vi "ExecuteState.vi"(0 "JSONRPC Server in":refnum<class "JSONRPC Server.lvclass">, 1 "IFw session":refnum<class "niInstr FIFO Register Bus v1 Host.lvclass">, 2 "FPGA Ref":refnum<k20>, 5 "Parameters":T4, 7 "StateIn":T1, 11 "error in (no error)":errorcluster) -> (8 "StateOut":T1, 15 "error out":errorcluster)   [LabVIEW 2017, in "AppStateMachine runtime.lvclass"]
uses:
  AppStateMachine runtime.lvclass
  <vilib>/NI/NI JSONRPC Server Framework/Classes/Server/JSONRPC Server.lvclass
  parameter user data.ctl
  <instrlib>/_niInstr/FIFO Register Bus/v1/Host/niInstr FIFO Register Bus v1 Host.lvclass
  State.ctl
  StateId.ctl
  LED_Color.ctl
  FPGA/FPGAtypedef.ctl
  Support/methods.ctl
  <vilib>/NI/NI JSONRPC Server Framework/Classes/Request/Request.lvclass/Request.ctl
  Responses/ResouceUsage.ctl
  <vilib>/NI/JSON Support for LabVIEW/JSON Data Classes/JSON Datatype/JSON Null.lvclass
  <vilib>/NI/NI JSONRPC Server Framework/Classes/Request/Read method.vi
  <vilib>/NI/NI JSONRPC Server Framework/Classes/Request/Read params.vi
  <vilib>/NI/JSON Support for LabVIEW/JSON Data Classes/JSON String/JSON String.lvclass
  C:/Program Files (x86)/National Instruments/LabVIEW 2017/vi.lib/NI/JSON Support for LabVIEW/JSON Data Classes/JSON Datatype/JSON Null.lvclass
  <vilib>/NI/JSON Support for LabVIEW/JSON Data Classes/JSON Array/JSON Array.lvclass
  <vilib>/NI/NI JSONRPC Server Framework/Classes/Server/Add Response (Result from Request).vi
  <vilib>/NI/JSON Support for LabVIEW/JSON Data Classes/JSON String/New JSON String.vi
  <vilib>/NI/JSON Support for LabVIEW/JSON Data Classes/JSON Array/New JSON Array (String).vi
  <vilib>/NI/JSON Support for LabVIEW/JSON Data Classes/JSON Array/New JSON Array (JSON Data).vi
  <vilib>/Utility/error.llb/Error Cluster From Error Code.vi
  <vilib>/rvi/errors/niLvFpgaAdjustHostInterfaceError.vi
  <vilib>/rvi/interface/nirviReadWriteControl/nirviReadWriteControl.xnode
  <vilib>/NI/NI JSONRPC Server Framework/Classes/Request/Request.lvclass
  <vilib>/NI/NI JSONRPC Server Framework/Classes/params/params.lvclass
  NiFpgaLv.dll
  <vilib>/rvi/interface/Simulation/niFpgaSimulationCallBeginRW.vi
  <vilib>/NI/JSON Support for LabVIEW/JSON Data Classes/JSON Helper/JSON Helper.lvclass
  C:/Program Files (x86)/National Instruments/LabVIEW 2017/vi.lib/NI/JSON Support for LabVIEW/JSON Data Classes/JSON Basic Type/JSON Literal.lvclass
  C:/Program Files (x86)/National Instruments/LabVIEW 2017/vi.lib/NI/JSON Support for LabVIEW/JSON Data Classes/JSON Structured Type/JSON Structure.lvclass
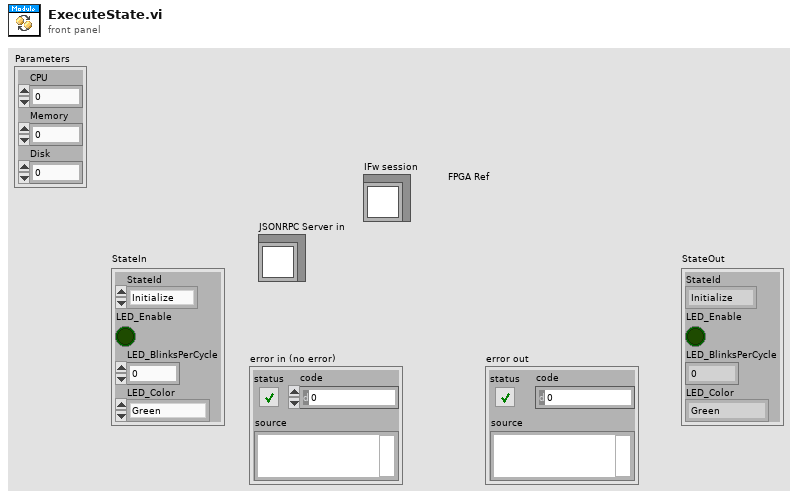
[diagram p1: front panel]
types:
  T1 = typedef "AppStateMachine runtime.lvclass/State.ctl" = cluster{"StateId":T2, "LED_Enable":bool, "LED_BlinksPerCycle":i32, "LED_Color":T3}
  T2 = typedef "AppStateMachine runtime.lvclass/StateId.ctl" = enum16{"Initialize", "Idle", "SafeState", "UnrecoverableSafeState"}
  T3 = typedef "AppStateMachine runtime.lvclass/LED_Color.ctl" = enum16{"Green", "Yellow"}
  T4 = typedef "AppStateMachine runtime.lvclass/parameter user data.ctl" = cluster{"CPU":dbl, "Memory":dbl, "Disk":dbl}
  T5 = typedef "AppStateMachine runtime.lvclass/methods.ctl" = enum16{"none", "echo", "GetResourceUsage", "CheckConnection", "CurrentState", "GoToSafeState", "ClearSafeState", "AvailableLogs", "ForceLogTrigger"}
  T6 = typedef "AppStateMachine runtime.lvclass/FPGAtypedef.ctl" = refnum<k20>
  T7 = typedef "AppStateMachine runtime.lvclass/ResouceUsage.ctl" = cluster{"CPU":dbl, "Memory":dbl, "Disk":dbl}
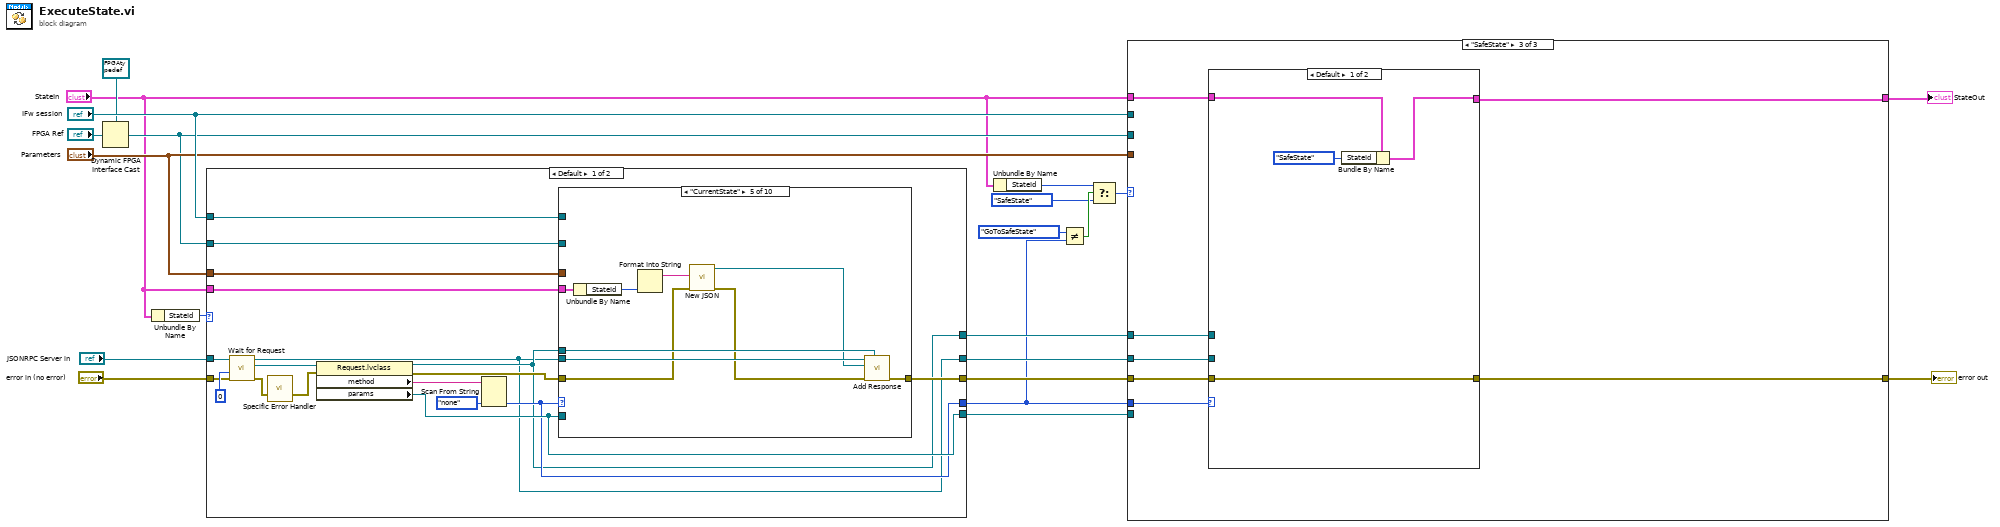
[diagram p0: block diagram]
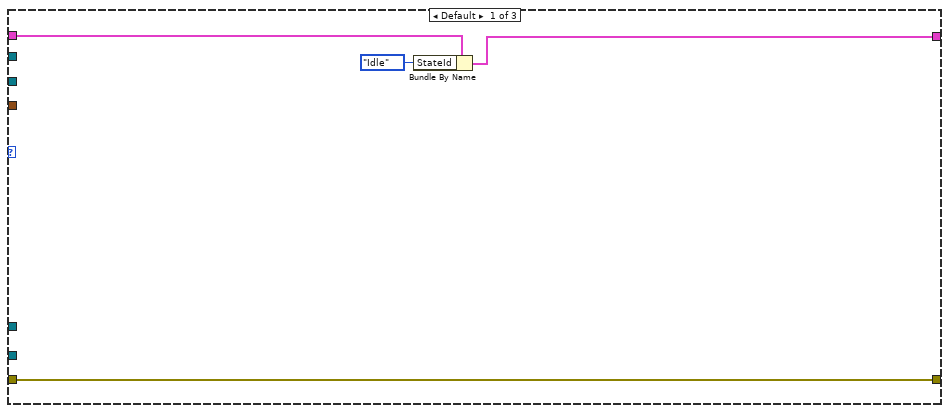
[diagram p2: hidden frame]
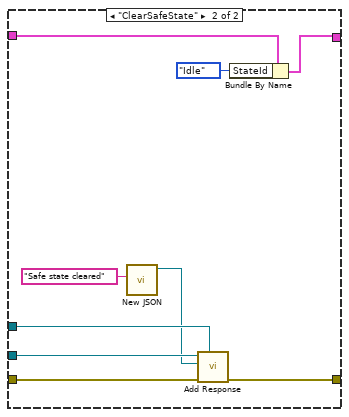
[diagram p4: hidden frame]
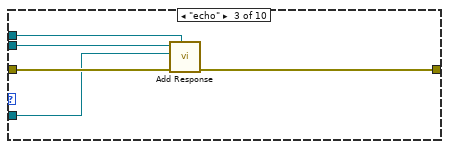
[diagram p7: hidden frame]
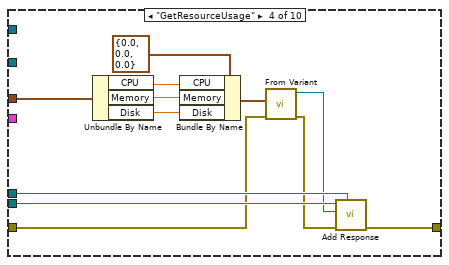
[diagram p8: hidden frame]
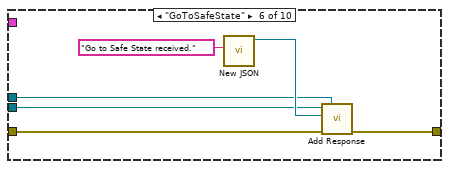
[diagram p9: hidden frame]
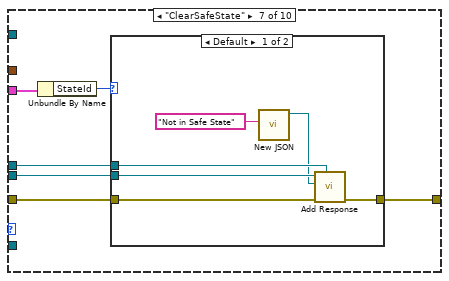
[diagram p10: hidden frame]
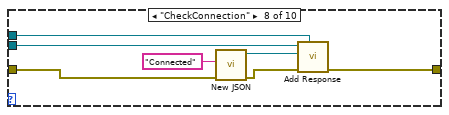
[diagram p12: hidden frame]
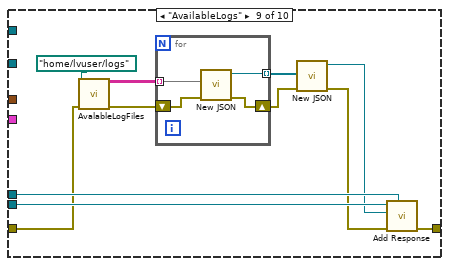
[diagram p13: hidden frame]
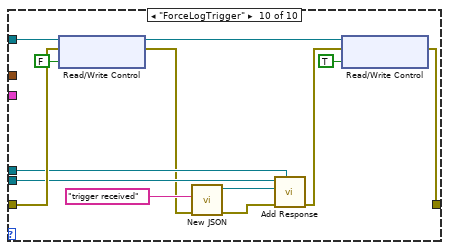
[diagram p14: hidden frame]
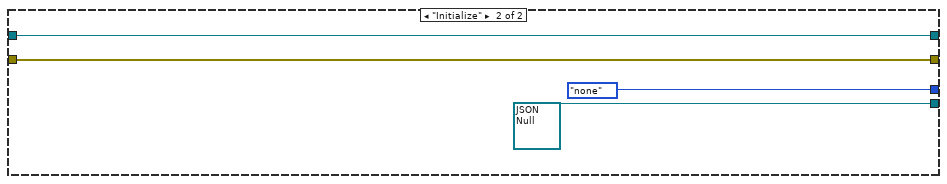
[diagram p15: hidden frame]
diagram:
  n1 = Dynamic FPGA Interface Cast(Session In=T6 refnum ("FPGA typedef"), Type="FPGA Ref") -> (Session Out=w11:T6)
  n2 = Unbundle By Name("StateIn") -> ("StateId"=w8:T2)
  n3 = case shown="Default" w8 {
    tunnel: "JSONRPC Server in" -> [w39 w124]
    tunnel: [w23 _] -> w21
    tunnel: "error in (no error)" -> [w37 w125]
    tunnel: [w28 w125] -> w20
    tunnel: [w22 w124] -> w16
    tunnel: [w25 refnum<class "JSON Null.lvclass"> refnum ("params")] -> w15
    tunnel: "IFw session" -> [w30 _]
    tunnel: w11 -> [w31 _]
    tunnel: [w24 methods."none" ("methods")] -> w6
    tunnel: "Parameters" -> [w29 _]
    tunnel: "StateIn" -> [w26 _]
    frame Default {
      n4 = call <vilib>:"Wait for Request.vi"("error in (no error)"=w37, "timeout in ms (100)"=0, "Server in"=w39) -> ("error out"=w36:errorcluster, "Request"=w35:refnum<class "Request.lvclass">, "Server out"=w22:refnum<class "JSONRPC Server.lvclass">)  [unwired: 5 in, 1 out]
      n5 = call "Specific Error Handler"("Error to Check"=w36) -> ("error out"=w34:errorcluster)  [unwired: 11 in, 3 out]
      n6 = property class="Request.lvclass"(reference=w35, error in=w34) -> (reference out=w23:refnum<class "Request.lvclass">, error out=w32:errorcluster, "method"=w27:string, "params"=w25:refnum<class "JSON Null.lvclass">)
      n7 = Scan From String(input string=w27, default 1=methods."none" ("methods")) -> (output 1=w24:T5)  [unwired: 3 in, 3 out]
      n8 = case shown="\"CurrentState\"" w24 {
        tunnel: w25 -> [_ _ w42 _ _ _ _ _ _ _]
        tunnel: w32 -> [w40 w41 w44 w48 w61 w73 w77 w89 w101 w120]
        tunnel: w23 -> [_ _ w45 w52 w66 w68 w75 w92 w102 w119]
        tunnel: w22 -> [_ _ w46 w51 w65 w69 w74 w91 w103 w118]
        tunnel: w31 -> [_ _ _ _ _ _ _ _ _ w121]
        tunnel: w30 -> [_ _ _ _ _ _ _ _ _ _]
        tunnel: w29 -> [_ _ _ w58 _ _ _ _ _ _]
        tunnel: [w40 w41 w43 w53 w67 w72 w76 w93 w104 w113] -> w28
        tunnel: w26 -> [_ _ _ _ w64 _ w79 _ _ _]
        frame Default {
        }
        frame "none" {
        }
        frame "echo" {
          n9 = call-poly <vilib>:"Add Response.vi"("Request"=w45, "error in (no error)"=w44, "JSON in"=w42, "Server in"=w46) -> ("error out"=w43:errorcluster)  [unwired: 5 in, 2 out]
        }
        frame "GetResourceUsage" {
          n10 = Unbundle By Name(w58) -> ("CPU"=w56:dbl, "Memory"=w55:dbl, "Disk"=w54:dbl)
          n11 = Bundle By Name(cluster=T7 {"CPU"=0.0, "Memory"=0.0, "Disk"=0.0} ("ResourceUsage"), "CPU"=w56, "Memory"=w55, "Disk"=w54) -> (w50:T7)
          n12 = call <vilib>:"From Variant.vi"("error in (no error)"=w48, "Variant"=w50) -> ("error out"=w47:errorcluster, "JSON out"=w49:refnum<class "JSON Null.lvclass">)  [unwired: 8 in]
          n13 = call-poly <vilib>:"Add Response.vi"("Request"=w52, "error in (no error)"=w47, "JSON in"=w49, "Server in"=w51) -> ("error out"=w53:errorcluster)  [unwired: 5 in, 2 out]
        }
        frame "CurrentState" {
          n14 = Unbundle By Name(w64) -> ("StateId"=w63:T2)
          n15 = Format Into String(w63) -> (resulting string=w62:string)  [unwired: 3 in, 1 out]
          n16 = call-poly <vilib>:"New JSON.vi"("error in (no error)"=w61, "value"=w62) -> ("error out"=w59:errorcluster, "JSON String out"=w60:refnum<class "JSON String.lvclass">)  [unwired: 8 in]
          n17 = call-poly <vilib>:"Add Response.vi"("Request"=w66, "error in (no error)"=w59, "JSON in"=w60, "Server in"=w65) -> ("error out"=w67:errorcluster)  [unwired: 5 in, 2 out]
        }
        frame "GoToSafeState" {
          n18 = call-poly <vilib>:"New JSON.vi"("value"="Go to Safe State received.") -> ("JSON String out"=w70:refnum<class "JSON String.lvclass">)  [unwired: 9 in, 1 out]
          n19 = call-poly <vilib>:"Add Response.vi"("Request"=w68, "error in (no error)"=w73, "JSON in"=w70, "Server in"=w69) -> ("error out"=w72:errorcluster)  [unwired: 5 in, 2 out]
        }
        frame "ClearSafeState" {
          n20 = Unbundle By Name(w79) -> ("StateId"=w78:T2)
          n21 = case shown="Default" w78 {
            tunnel: w77 -> [w84 w86]
            tunnel: [w85 w86] -> w76
            tunnel: w75 -> [w83 _]
            tunnel: w74 -> [w82 _]
            frame Default {
              n22 = call-poly <vilib>:"New JSON.vi"("value"="Not in Safe State" ("String")) -> ("JSON String out"=w80:refnum<class "JSON String.lvclass">)  [unwired: 9 in, 1 out]
              n23 = call-poly <vilib>:"Add Response.vi"("Request"=w83, "error in (no error)"=w84, "JSON in"=w80, "Server in"=w82) -> ("error out"=w85:errorcluster)  [unwired: 5 in, 2 out]
            }
            frame "SafeState" {
            }
          }
        }
        frame "CheckConnection" {
          n24 = call-poly <vilib>:"New JSON.vi"("error in (no error)"=w89, "value"="Connected" ("String")) -> ("error out"=w87:errorcluster, "JSON String out"=w88:refnum<class "JSON String.lvclass">)  [unwired: 8 in]
          n25 = call-poly <vilib>:"Add Response.vi"("Request"=w92, "error in (no error)"=w87, "JSON in"=w88, "Server in"=w91) -> ("error out"=w93:errorcluster)  [unwired: 5 in, 2 out]
        }
        frame "AvailableLogs" {
          n26 = call "AvalableLogFiles.vi"("path"=path "/home/lvuser/logs", "error in (no error)"=w101) -> ("FilesInfo"=w99:string[][], "error out"=w98:errorcluster)  [unwired: 12 in]
          n27 = for {
            tunnel: w99 -> [w108] mode=indexing
            shift-right: [w106] -> w96
            shift-left: w98 -> [w107]
            tunnel: [w105] -> w97 mode=indexing
            n28 = call-poly <vilib>:"New JSON.vi"("error in (no error)"=w107, "String Array"=w108) -> ("error out"=w106:errorcluster, "JSON Array out"=w105:refnum<class "JSON Array.lvclass">)  [unwired: 8 in]
          }
          n29 = call-poly <vilib>:"New JSON.vi"("error in (no error)"=w96, "JSON Datatypes"=w97) -> ("error out"=w95:errorcluster, "JSON Array out"=w94:refnum<class "JSON Array.lvclass">)  [unwired: 8 in]
          n30 = call-poly <vilib>:"Add Response.vi"("Request"=w102, "error in (no error)"=w95, "JSON in"=w94, "Server in"=w103) -> ("error out"=w104:errorcluster)  [unwired: 5 in, 2 out]
        }
        frame "ForceLogTrigger" {
          n31 = xnode "Read/Write Control"("FPGA VI Reference In"=w121, "error in"=w120, "ManualTrigger"=FALSE) -> ("FPGA VI Reference Out"=w116:T6, "error out"=w110:errorcluster)
          n32 = call-poly <vilib>:"New JSON.vi"("error in (no error)"=w110, "value"="trigger received" ("String")) -> ("error out"=w109:errorcluster, "JSON String out"=w112:refnum<class "JSON String.lvclass">)  [unwired: 8 in]
          n33 = call-poly <vilib>:"Add Response.vi"("Request"=w119, "error in (no error)"=w109, "JSON in"=w112, "Server in"=w118) -> ("error out"=w114:errorcluster)  [unwired: 5 in, 2 out]
          n34 = xnode "Read/Write Control"("FPGA VI Reference In"=w116, "error in"=w114, "ManualTrigger"=TRUE) -> ("error out"=w113:errorcluster)  [unwired: 1 out]
        }
      }
    }
    frame "Initialize" {
    }
  }
  n35 = Unbundle By Name("StateIn") -> ("StateId"=w3:T2)
  n36 = Not Equal?(x=methods."GoToSafeState", y=w6) -> (x != y?=w2:bool)
  n37 = Select(t=w3, s=w2, f=StateId."SafeState") -> (s? t:f=w4:T2)
  n38 = case shown="\"SafeState\"" w4 {
    tunnel: w20 -> [w129 w131 w137]
    tunnel: w21 -> [_ _ w135]
    tunnel: [w129 w131 w132] -> w17
    tunnel: w16 -> [_ _ w136]
    tunnel: w15 -> [_ _ _]
    tunnel: w6 -> [_ _ w138]
    tunnel: "IFw session" -> [_ _ _]
    tunnel: w11 -> [_ _ _]
    tunnel: "Parameters" -> [_ _ _]
    tunnel: "StateIn" -> [w128 w130 w134]
    tunnel: [w126 w130 w133] -> w7
    frame Default {
      n39 = Bundle By Name(cluster=w128, "StateId"=StateId."Idle") -> (w126:T1)
    }
    frame "Idle" {
    }
    frame "SafeState" {
      n40 = case shown="Default" w138 {
        tunnel: w137 -> [w142 w151]
        tunnel: w136 -> [_ w150]
        tunnel: w135 -> [_ w149]
        tunnel: w134 -> [w140 w146]
        tunnel: [w139 w144] -> w133
        tunnel: [w142 w143] -> w132
        frame Default {
          n41 = Bundle By Name(cluster=w140, "StateId"=StateId."SafeState") -> (w139:T1)
        }
        frame "ClearSafeState" {
          n42 = call-poly <vilib>:"New JSON.vi"("value"="Safe state cleared") -> ("JSON String out"=w147:refnum<class "JSON String.lvclass">)  [unwired: 9 in, 1 out]
          n43 = call-poly <vilib>:"Add Response.vi"("Request"=w149, "error in (no error)"=w151, "JSON in"=w147, "Server in"=w150) -> ("error out"=w143:errorcluster)  [unwired: 5 in, 2 out]
          n44 = Bundle By Name(cluster=w146, "StateId"=StateId."Idle") -> (w144:T1)
        }
      }
    }
  }
  "error out" <- w17
  "StateOut" <- w7
